vi "Single SSC DCPower Configure Single Point Force DC Voltage Asymmetric Limits.vi"(0 "DCPower SSC in":T1, 1 "Voltage Level Range (V)":dbl format="%#_6p", 2 "Current Limit Range (A)":dbl format="%#_6p", 5 "Voltage Level (V)":dbl format="%#_6p", 7 "Current Limit High (A)":dbl format="%#_6p", 9 "Current Limit Low (A)":dbl format="%#_6p", 11 "error in":errorcluster) -> (4 "DCPower SSC out":T1, 15 "error out":errorcluster)   [LabVIEW 2020]
doc: "This VI configures the instrument sessions to force a single voltage with asymmetric current limits."
uses:
  SSC DCPower.ctl
  <instrlib>/niDCPower/nidcpower.llb/niDCPower Source Mode.ctl
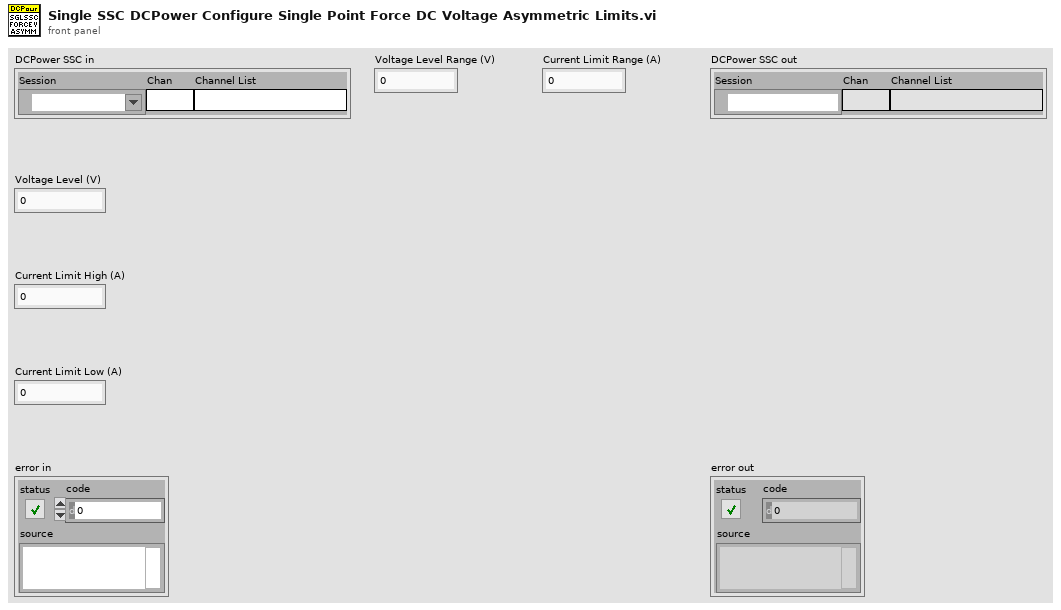
[diagram p1: front panel]
types:
  T1 = typedef "SSC DCPower.ctl" = cluster{"Session":refnum<k15>, "Chan":string, "Channel List":string}
  T2 = typedef "niDCPower Source Mode.ctl" = i32
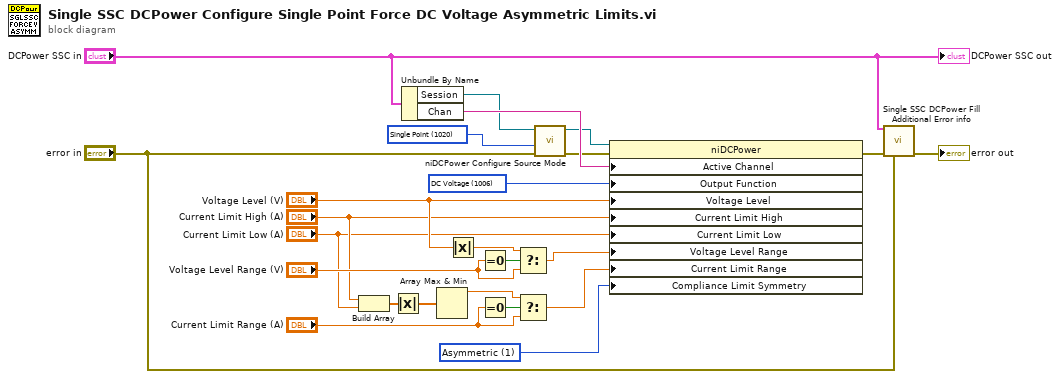
[diagram p0: block diagram]
diagram:
  w5 = 1 items=["Symmetric", "Asymmetric"] ("Source:Advanced:Compliance Limit Symmetry")
  w9 = T2 1020 items=["Single Point"=1020, "Sequence"=1021] ("source mode")
  w13 = 1006 items=["DC Voltage"=1006, "DC Current"=1007, "Pulse Voltage"=1049, "Pulse Current"=1050] ("Source:Output Function")
  n1 = Build Array("Current Limit High (A)", "Current Limit Low (A)") -> (w2:dbl[])
  n2 = Absolute Value(x=w2) -> (abs(x)=w17:dbl[])
  n3 = Unbundle By Name("DCPower SSC in") -> ("Session"=w11:refnum<k15>, "Chan"=w14:string)
  n4 = Array Max & Min(array=w17) -> (max value=w1:dbl)  [unwired: 3 out]
  n5 = Absolute Value(x="Voltage Level (V)") -> (abs(x)=w20:dbl)
  n6 = Equal To 0?(x="Voltage Level Range (V)") -> (x = 0?=w19:bool)
  n7 = Equal To 0?(x="Current Limit Range (A)") -> (x = 0?=w18:bool)
  n8 = Select(t=w20, s=w19, f="Voltage Level Range (V)") -> (s? t:f=w16:dbl)
  n9 = Select(t=w1, s=w18, f="Current Limit Range (A)") -> (s? t:f=w15:dbl)
  n10 = call <instrlib>:"niDCPower Configure Source Mode.vi"("error in (no error)"="error in", "source mode"=w9, "instrument handle"=w11) -> ("error out"=w12:errorcluster, "instrument handle out"=w10:refnum<k15>)  [unwired: 7 in]
  n11 = property class="niDCPower"(reference=w10, error in=w12, "Active Channel"=w14, "Output Function"=w13, "Voltage Level"="Voltage Level (V)", "Current Limit High"="Current Limit High (A)", "Current Limit Low"="Current Limit Low (A)", "Voltage Level Range"=w16, "Current Limit Range"=w15, "Compliance Limit Symmetry"=w5) -> (error out=w24:errorcluster)  [unwired: 1 out]
  n12 = call "Single SSC DCPower Fill Additional Error info.vi"("DCPower SSC in"="DCPower SSC in", "error in"=w24, "previous error in"="error in") -> ("error out"=→"error out":errorcluster)  [unwired: 12 in]
  "DCPower SSC out" <- "DCPower SSC in"
